vi "SV TDMS Write DBL Array (1 Ch).vi"(0 "tdms file":refnum<k34>, 1 "write properties (T)":bool, 5 "group name in":string="Waveform", 7 "channel name in":string, 9 "scaled signal [EU]":dbl[](array[numeric]), 11 "error in":errorcluster, 12 "channel description":string, 13 "unit label":string) -> (4 "tdms file out":refnum<k34>, 6 "group name out":string="Waveform", 8 "channel name out":string, 15 "error out":errorcluster)   [LabVIEW 2017]
uses:
  <vilib>/addons/_NISVFA/_Shared subVIs/Controls/LV Datatypes.ctl
  <vilib>/addons/_NISVFA/_Shared subVIs/Controls/NI Channel Properties.ctl
  <vilib>/addons/_NISVFA/_Shared subVIs/Controls/svc_X-Axis Units.ctl
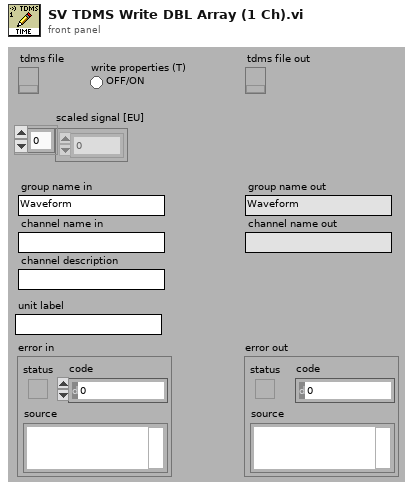
[diagram p1: front panel]
types:
  T1 = typedef "svc_X-Axis Units.ctl" = u16
  T2 = typedef "NI Channel Properties.ctl" = u16
  T3 = typedef "LV Datatypes.ctl" = i32
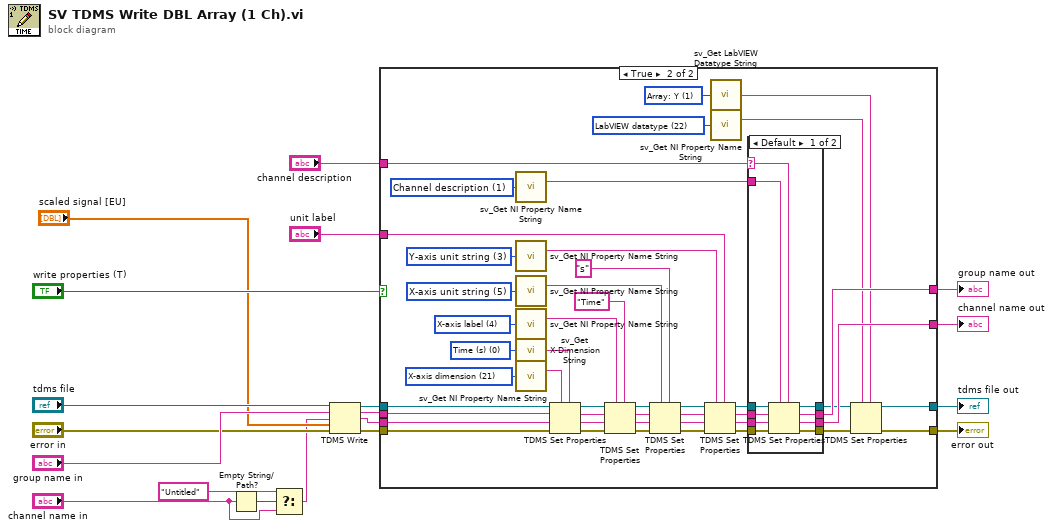
[diagram p0: block diagram]
diagram:
  n1 = Empty String/Path?(string/path="channel name in") -> (empty?=w4:bool)
  n2 = Select(t="Untitled" ("channel name"), s=w4, f="channel name in") -> (s? t:f=w2:string)
  n3 = TDMS Write(0:"tdms file", 5:"group name in", 7:w2, 9:"scaled signal [EU]", 11:"error in") -> (4:w10:refnum<k34>, 6:w15:string, 8:w16:string, 15:w14:errorcluster)  [unwired: 1 in]
  n4 = case shown="True" "write properties (T)" {
    tunnel: "channel description" -> [_ w69]
    tunnel: [w22 w45] -> w18
    tunnel: [w23 w44] -> w17
    tunnel: "unit label" -> [_ w60]
    tunnel: w16 -> [w20 w42]
    tunnel: w15 -> [w21 w41]
    tunnel: w14 -> [w23 w43]
    tunnel: w10 -> [w22 w40]
    tunnel: [w21 w53] -> w9
    tunnel: [w20 w52] -> w8
    frame False {
    }
    frame True {
      w25 = T1 0 items=["Time (s)"=0, "Frequency-CB (Hz)"=1, "Frequency-CPB (Hz)"=1248, "Frequency-Arbitrary (Hz)"=2357, "Quefrency (s)"=2, "Revolutions (rev)"=3, "Order"=4, "Speed (RPM)"=11, "Speed (rad/s)"=21, "Index"=65535] ("x-axis units")
      w27 = T2 1 items=["Channel name", "Channel description", "Y-axis label", "Y-axis unit string", "X-axis label", "X-axis unit string", "x0", "dx", "Number of samples", "X channel", "Filter settled", "dB reference", "Window", "Window parameter", "Window size", "FFT size", "Peak units", "Spectrum type", "Magnitude scale", "Spectral density", "Sensor sensitivity (mV/EU)", "X-axis dimension", "LabVIEW datatype", "Function type", "Function subtype"] ("property")
      w29 = T2 3 items=["Channel name", "Channel description", "Y-axis label", "Y-axis unit string", "X-axis label", "X-axis unit string", "x0", "dx", "Number of samples", "X channel", "Filter settled", "dB reference", "Window", "Window parameter", "Window size", "FFT size", "Peak units", "Spectrum type", "Magnitude scale", "Spectral density", "Sensor sensitivity (mV/EU)", "X-axis dimension", "LabVIEW datatype", "Function type", "Function subtype"] ("property")
      w37 = T2 5 items=["Channel name", "Channel description", "Y-axis label", "Y-axis unit string", "X-axis label", "X-axis unit string", "x0", "dx", "Number of samples", "X channel", "Filter settled", "dB reference", "Window", "Window parameter", "Window size", "FFT size", "Peak units", "Spectrum type", "Magnitude scale", "Spectral density", "Sensor sensitivity (mV/EU)", "X-axis dimension", "LabVIEW datatype", "Function type", "Function subtype"] ("property")
      w38 = T2 4 items=["Channel name", "Channel description", "Y-axis label", "Y-axis unit string", "X-axis label", "X-axis unit string", "x0", "dx", "Number of samples", "X channel", "Filter settled", "dB reference", "Window", "Window parameter", "Window size", "FFT size", "Peak units", "Spectrum type", "Magnitude scale", "Spectral density", "Sensor sensitivity (mV/EU)", "X-axis dimension", "LabVIEW datatype", "Function type", "Function subtype"] ("property")
      w39 = T2 21 items=["Channel name", "Channel description", "Y-axis label", "Y-axis unit string", "X-axis label", "X-axis unit string", "x0", "dx", "Number of samples", "X channel", "Filter settled", "dB reference", "Window", "Window parameter", "Window size", "FFT size", "Peak units", "Spectrum type", "Magnitude scale", "Spectral density", "Sensor sensitivity (mV/EU)", "X-axis dimension", "LabVIEW datatype", "Function type", "Function subtype"] ("property")
      w51 = T2 22 items=["Channel name", "Channel description", "Y-axis label", "Y-axis unit string", "X-axis label", "X-axis unit string", "x0", "dx", "Number of samples", "X channel", "Filter settled", "dB reference", "Window", "Window parameter", "Window size", "FFT size", "Peak units", "Spectrum type", "Magnitude scale", "Spectral density", "Sensor sensitivity (mV/EU)", "X-axis domain", "LabVIEW datatype"] ("property")
      w50 = T3 1 items=["String"=-2, "Boolean"=-1, "Scalar: y"=0, "Array: Y"=1, "Waveform: t0, dt, Y, variant"=2, "Cluster: x0, dx, Y"=3, "Cluster: X, Y"=4, "Waterfall"=5, "Colormap"=6] ("LabVIEW datatype")
      n5 = call <vilib>:"sv_Get NI Property Name String.vi"("property"=w27) -> ("TDMS property name"=w26:string)  [unwired: 13 in, 1 out]
      n6 = call <vilib>:"sv_Get NI Property Name String.vi"("property"=w29) -> ("TDMS property name"=w28:string)  [unwired: 13 in, 1 out]
      n7 = call <vilib>:"sv_Get NI Property Name String.vi"("property"=w37) -> ("TDMS property name"=w36:string)  [unwired: 13 in, 1 out]
      n8 = call <vilib>:"sv_Get NI Property Name String.vi"("property"=w38) -> ("TDMS property name"=w35:string)  [unwired: 13 in, 1 out]
      n9 = call <vilib>:"sv_Get X-Dimension String.vi"("x-axis units"=w25) -> ("x-domain string"=w24:string)  [unwired: 4 in]
      n10 = call <vilib>:"sv_Get NI Property Name String.vi"("property"=w39) -> ("TDMS property name"=w34:string)  [unwired: 13 in, 1 out]
      n11 = TDMS Set Properties(5:w24, 7:w34, 8:w43, 9:w42, 10:w41, 11:w40) -> (0:w30:errorcluster, 1:w31:string, 2:w32:string, 3:w33:refnum<k34>)
      n12 = TDMS Set Properties(5:"Time" ("channel name"), 7:w35, 8:w30, 9:w31, 10:w32, 11:w33) -> (0:w54:errorcluster, 1:w55:string, 2:w56:string, 3:w57:refnum<k34>)
      n13 = TDMS Set Properties(5:"s" ("group name"), 7:w36, 8:w54, 9:w55, 10:w56, 11:w57) -> (0:w62:errorcluster, 1:w63:string, 2:w64:string, 3:w61:refnum<k34>)
      n14 = TDMS Set Properties(5:w60, 7:w28, 8:w62, 9:w63, 10:w64, 11:w61) -> (0:w68:errorcluster, 1:w67:string, 2:w66:string, 3:w65:refnum<k34>)
      n15 = call <vilib>:"sv_Get LabVIEW Datatype String.vi"("LabVIEW datatype"=w50) -> ("datatype string"=w49:string)  [unwired: 4 in]
      n16 = call <vilib>:"sv_Get NI Property Name String.vi"("property"=w51) -> ("TDMS property name"=w48:string)  [unwired: 13 in, 1 out]
      n17 = case shown="Default" w69 {
        selector: w69 -> [w72 _]
        tunnel: w26 -> [w79 _]
        tunnel: w65 -> [w78 w83]
        tunnel: w66 -> [w77 w81]
        tunnel: w67 -> [w76 w80]
        tunnel: w68 -> [w75 w82]
        tunnel: [w74 w82] -> w46
        tunnel: [w73 w83] -> w47
        tunnel: [w71 w81] -> w53
        tunnel: [w70 w80] -> w52
        frame Default {
          n18 = TDMS Set Properties(5:w72, 7:w79, 8:w75, 9:w76, 10:w77, 11:w78) -> (0:w74:errorcluster, 1:w70:string, 2:w71:string, 3:w73:refnum<k34>)
        }
        frame "" {
        }
      }
      n19 = TDMS Set Properties(5:w49, 7:w48, 8:w46, 11:w47) -> (0:w44:errorcluster, 3:w45:refnum<k34>)  [unwired: 2 in, 2 out]
    }
  }
  "tdms file out" <- w18
  "error out" <- w17
  "channel name out" <- w8
  "group name out" <- w9
